vi "Spectrometer Control Panel (No Objects).vi"(8 "error in (no error)":errorcluster) -> (0 "error out":errorcluster)   [LabVIEW 2012]
uses:
  JY-SPEX-TRIAX/controls.llb/Turret Position (TRIAX).ctl
  JY-SPEX-TRIAX/controls.llb/Monochromator System Number.ctl
  JY-SPEX-TRIAX/controls.llb/Mirror Position.ctl
  Global/GPIB Type Def.ctl
  <vilib>/Utility/error.llb/DialogType.ctl
  JY-SPEX-TRIAX/controls.llb/Slits.ctl
  JY-SPEX-TRIAX/JY-SPEX-TRIAX.lvlib
panel:
  out "Shutter\nFunctional?":bool
  in  "JY Spectrometer":T1={"Name"="JY Spectrometer", "bus"=0.0, "GPIB"=1.0, "GPIB as string"="1", "byte"=1024, "VISA Resource Name"="GPIB0::1::INSTR"}
  out "Cluster Out":T5
  in  "Cluster In":T5
  out "?":bool
  out "Title 2":string="Spectrometer Control Program"
  in  "Select Grating":T4
  out "Construct":bool
  out "Init":T6
  out "Status":string
  in  "Shutter":bool
  in  "Set Mirror":bool
  in  "Exit Mirror Pos":bool=TRUE
  in  "Exit":bool
  out "Ready (when flashing)":bool
  out "Slits Open?":bool
  in  "Close Slits":bool
  in  "stepsize":dbl[unit]
  in  "Optimize":bool
  out "groovedensity":dbl[unit] caption="Groove Density"
  out "blazewave":dbl[unit] caption="Blaze Wavelength"
  in  "Set Turret":bool
  out "Title":string="Spectrometer Control Program"
  in  "Reset":bool
  out "Current Wavelength":dbl[unit]
  in  "Target Wavelength":dbl[unit]=4.0000000000000003e-07 min=0.0 max=1.4000000000000001e-06 step=1.0000000000000002e-10
  in  "Jump To Wavelength":bool
  in  "Set Slits":bool
  out "currentlat":dbl[unit] format="%#_6f"
  out "currentaxial":dbl[unit] format="%#_6f"
  in  "gotolat":dbl[unit] min=0.0 max=0.0022 step=1e-05
  in  "gotoaxial":dbl[unit] min=0.0 max=0.0022 step=1e-05 format="%#_6f"
  # "Initialization"
  # "Wavelength Control"
  # "Slit Widths"
  # "Turret and Other Specs"
  # "Target"
  # "Current"
  # "AXIAL/CCD"
  # "LATERAL/PMT"
  # "Axial Entrance"
  # "Lateral Exit"
  # "(will round to nearest step size - 2 µm)"
  # "Grooves/mm       Blaze           Cal Offset\nGrating A           1200           500 nm            -35571\nGrating B           1200           750 nm            -38317\nGrating C           Blank             N/A               -40000"
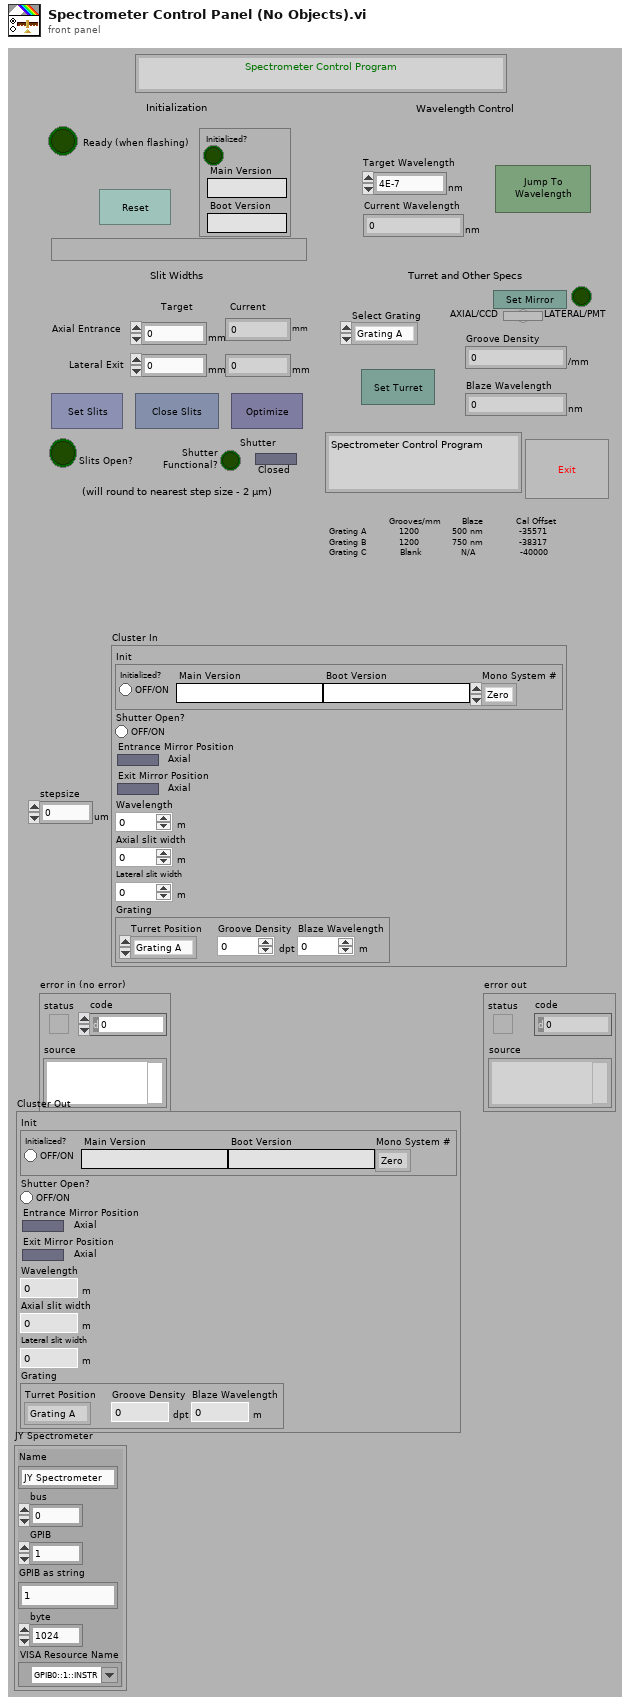
[diagram p1: front panel]
types:
  T1 = typedef "GPIB Type Def.ctl" = cluster{"Name":string, "bus":dbl, "GPIB":dbl, "GPIB as string":string, "byte":i32, "VISA Resource Name":refnum<visa-resource-name>}
  T2 = typedef "JY-SPEX-TRIAX.lvlib/Monochromator System Number.ctl" = enum16{"Zero", "One"}
  T3 = typedef "JY-SPEX-TRIAX.lvlib/Mirror Position.ctl" = bool
  T4 = typedef "JY-SPEX-TRIAX.lvlib/Turret Position (TRIAX).ctl" = enum16{"Grating A", "Grating B", "Grating C"}
  T5 = cluster{"Init":cluster{"Initialized?":bool, "Main Version":string, "Boot Version":string, "Mono System #":T2}, "Shutter Open?":bool, "Entrance Mirror Position":T3, "Exit Mirror Position":T3, "Wavelength":dbl[unit], "Axial slit width":dbl[unit], "Lateral slit width":dbl[unit], "Grating":cluster{"Turret Position":T4, "Groove Density":dbl[unit], "Blaze Wavelength":dbl[unit]}}
  T6 = cluster{"Initialized?":bool, "Main Version":string, "Boot Version":string, "Spectrometer Number":enum16{"Zero", "One"}}
  T7 = typedef "JY-SPEX-TRIAX.lvlib/Slits.ctl" = enum16{"0 (Front/Axial Entrance)", "1 (Side/Lateral Entrance)", "2 (Front/Axial Exit)", "3 (Side/Lateral Exit)"}
  T8 = typedef "DialogType.ctl" = u16
  T9 = cluster{"Initialized?":bool, "Main Version":string, "Boot Version":string, "Mono System #":T2}
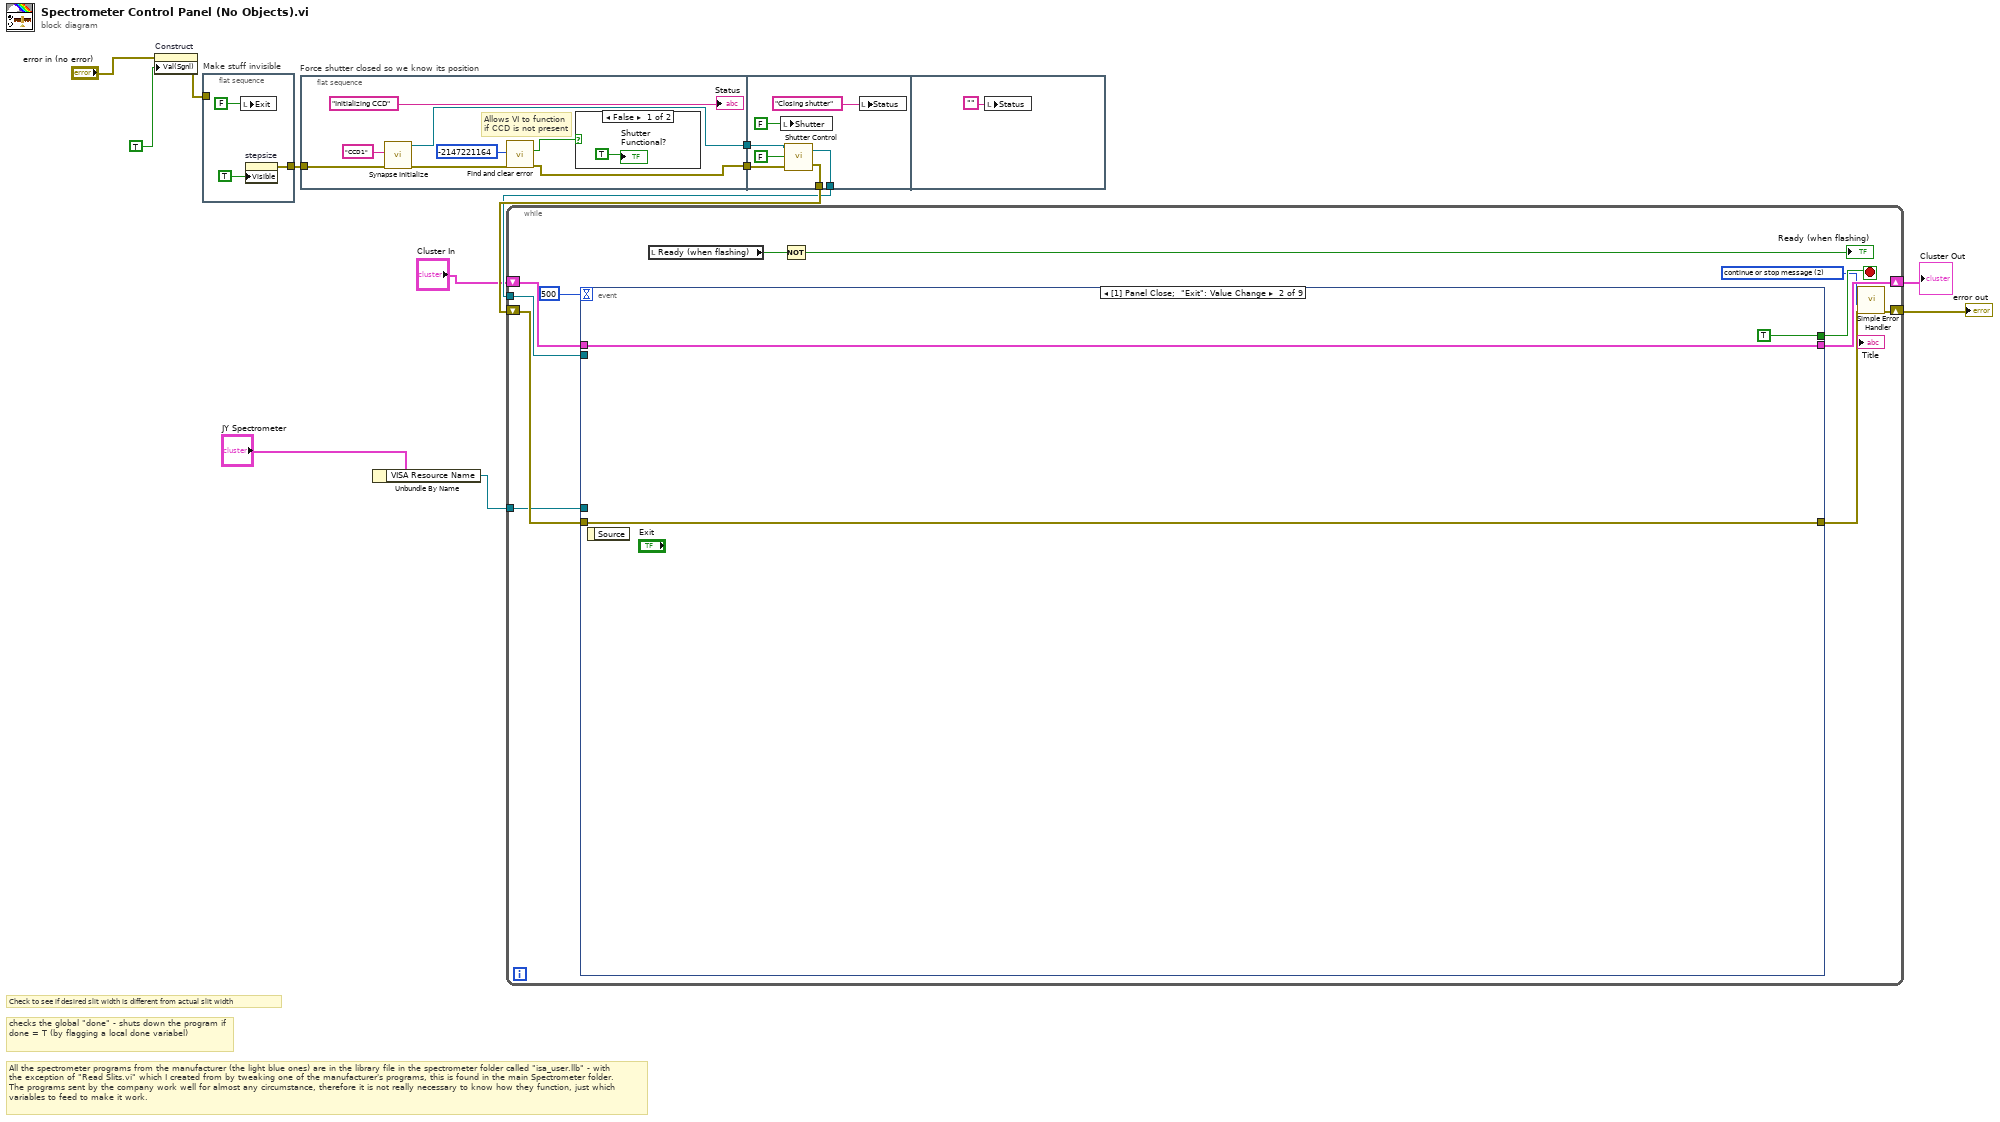
[diagram p0: block diagram]
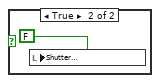
[diagram p2: hidden frame]
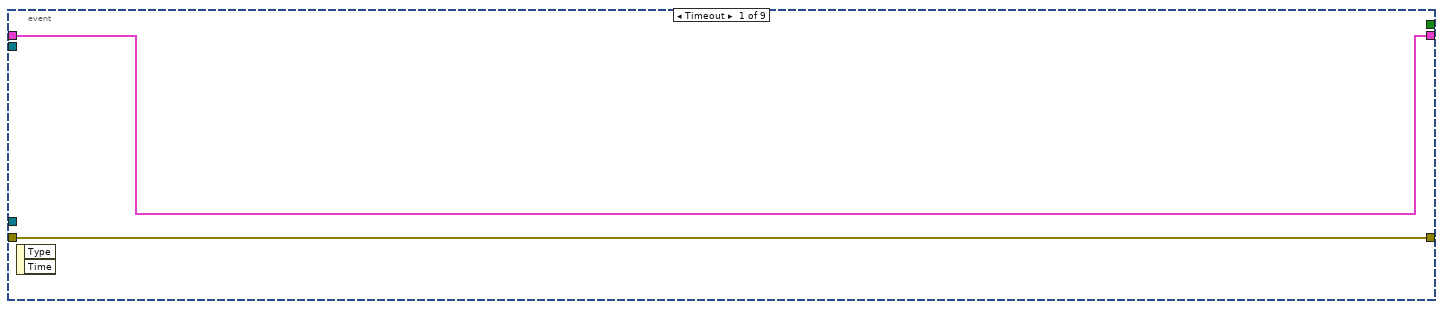
[diagram p3: hidden frame]
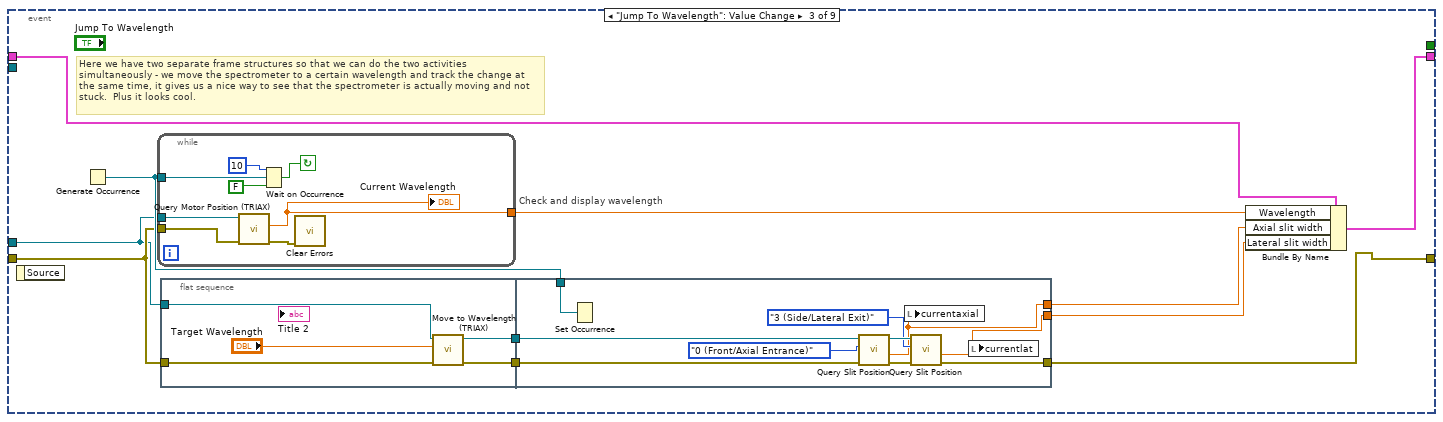
[diagram p4: hidden frame]
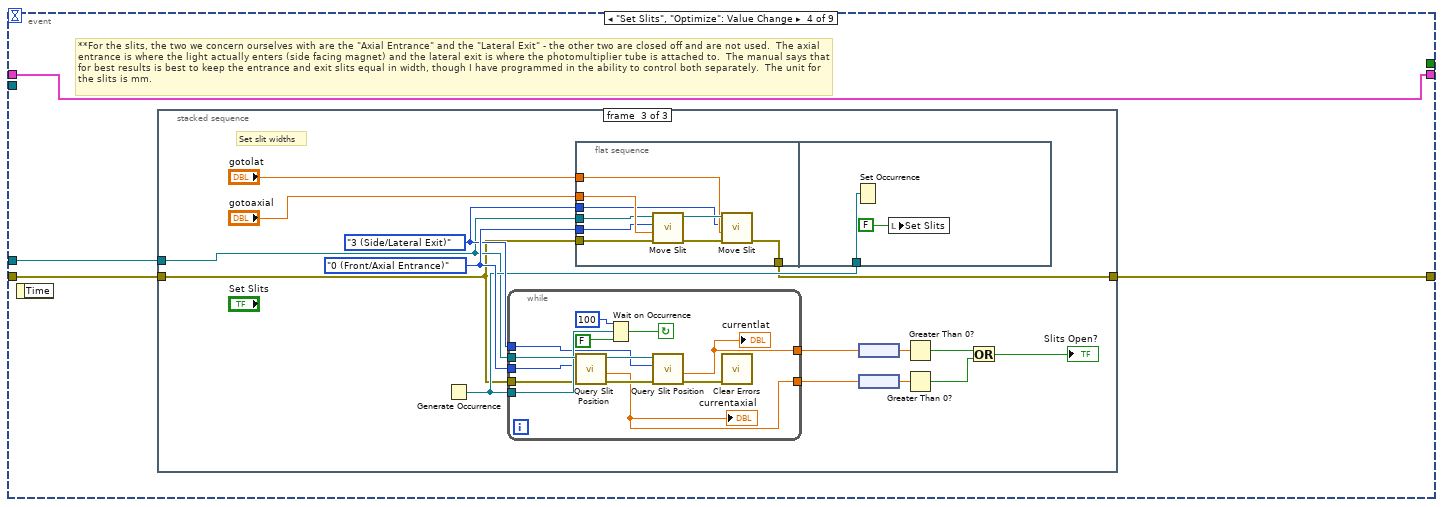
[diagram p5: hidden frame]
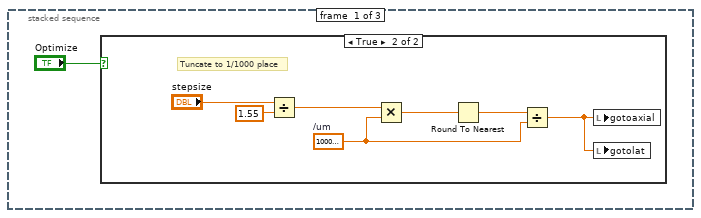
[diagram p6: hidden frame]
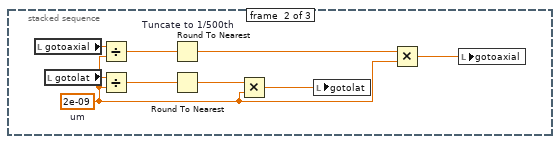
[diagram p8: hidden frame]
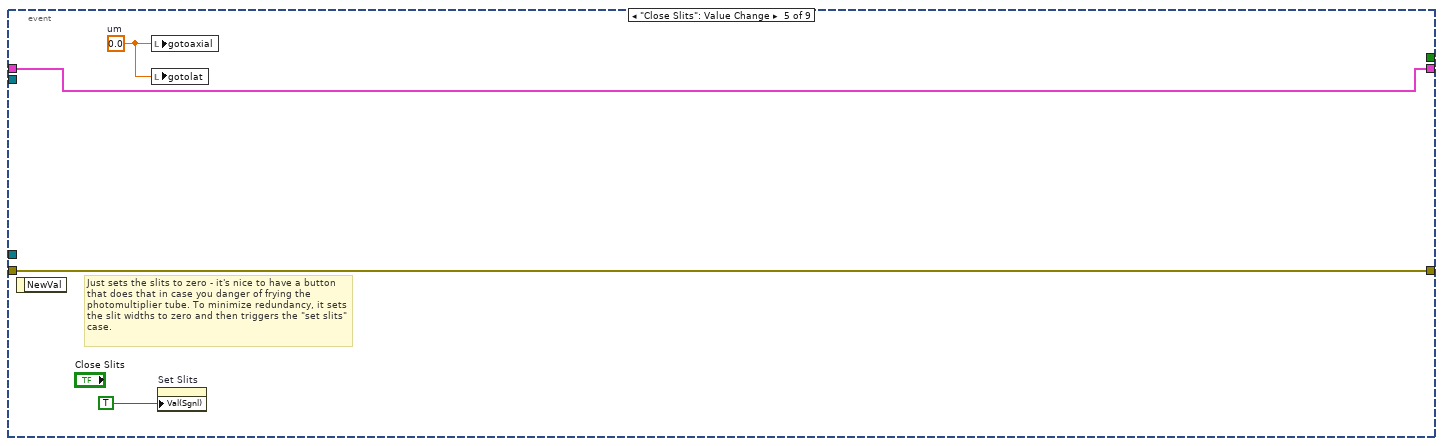
[diagram p9: hidden frame]
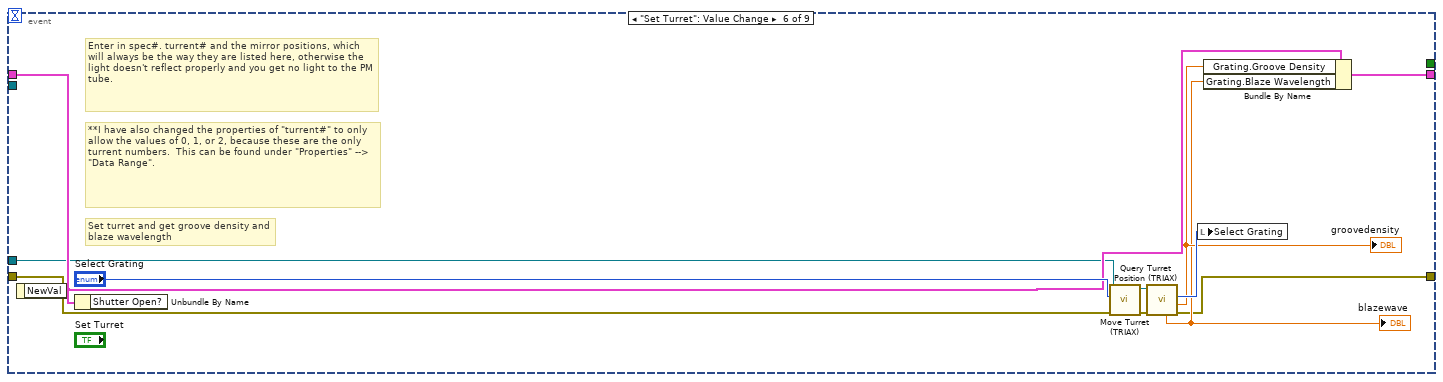
[diagram p10: hidden frame]
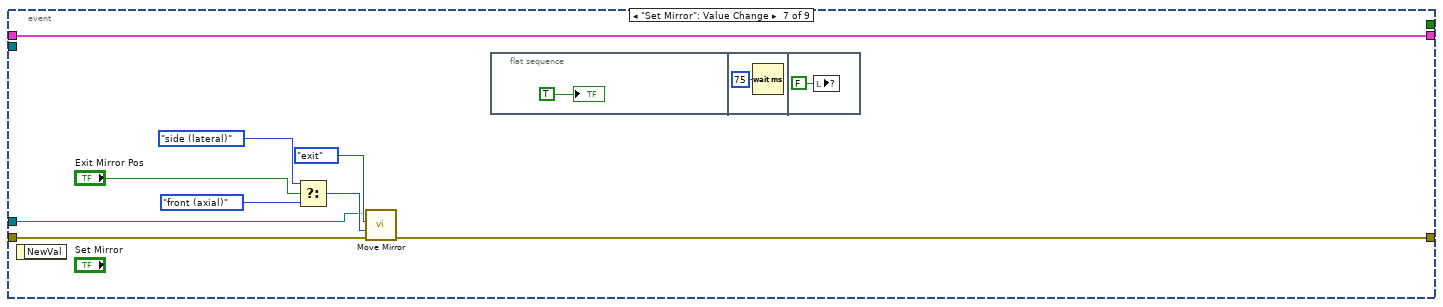
[diagram p11: hidden frame]
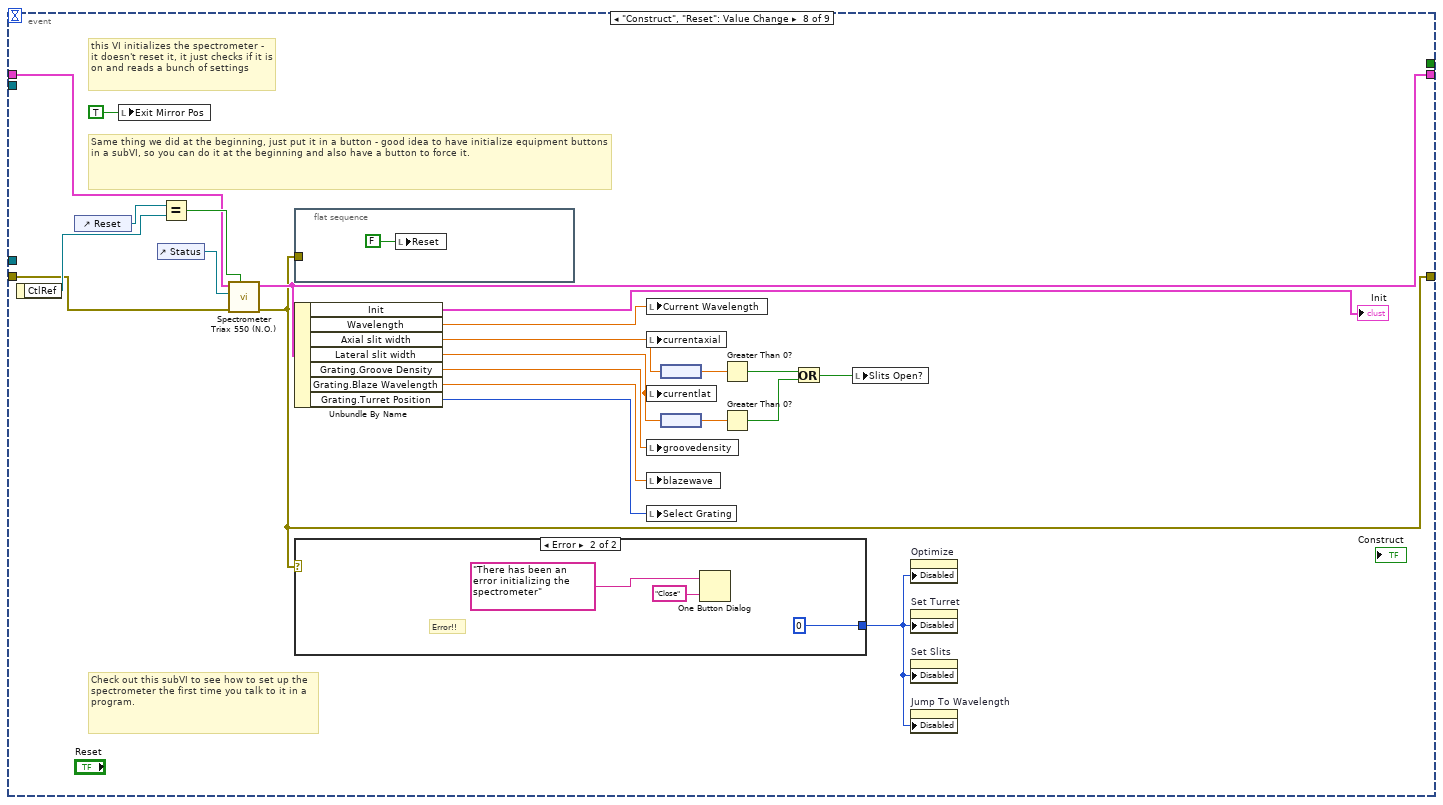
[diagram p12: hidden frame]
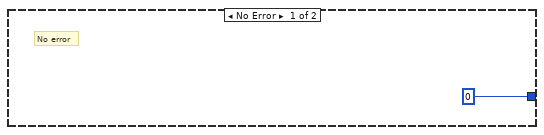
[diagram p13: hidden frame]
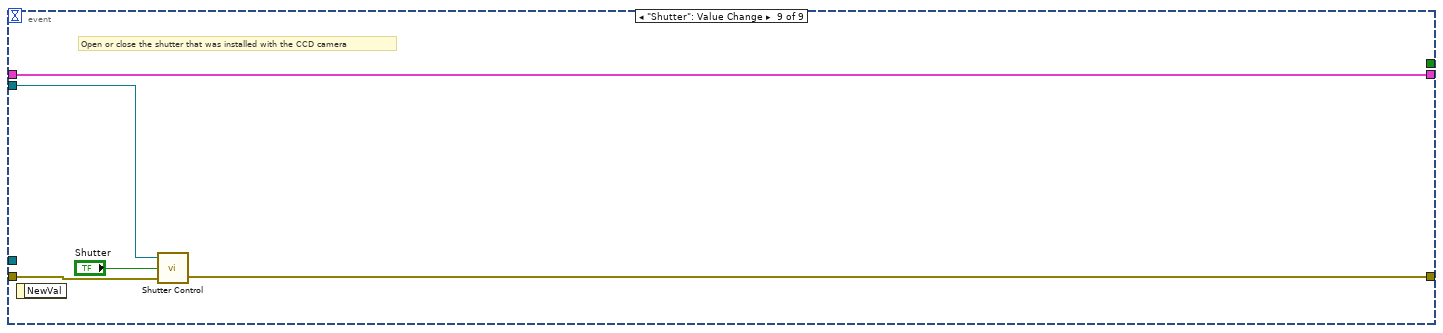
[diagram p14: hidden frame]
diagram:
  # "Check to see if desired slit width is different from actual slit width"
  # "checks the global \"done\" - shuts down the program if done = T (by flagging a local done variabel)"
  # "All the spectrometer programs from the manufacturer (the light blue ones) are in the library file in the spectrometer folder called \"isa_user.llb\" - with the exception of \"Read Slits.vi\" which I created from by tweaking one of the manufacturer's programs, this is found in the main Spectrometer folder.  The programs sent by the company work well for almost any circumstance, therefore it is not really necessary to know how they function, just which variables to feed to make it work."
  n1 = property on="Construct" class="Bool (strict)"(error in="error in (no error)", "Val(Sgnl)"=TRUE ("Value (Signaling)")) -> (error out=w12:errorcluster)  [unwired: 1 in, 1 out]
  n2 = flat-sequence "Make stuff invisible" {
    tunnel: w12 -> [_]
    tunnel: [w15] -> w9
    frame #0 {
      n3 = local write "Exit"(FALSE ("exit")) -> ()
      n4 = property on="stepsize" class="DigNum (strict)"("Visible"=TRUE) -> (error out=w15:errorcluster)  [unwired: 2 in, 1 out]
    }
  }
  n5 = flat-sequence "Force shutter closed so we know its position" {
    tunnel: w9 -> [w23]
    tunnel: [w18] -> w8
    tunnel: [w17] -> w1
    tunnel: [w31] -> w11
    tunnel: [w30] -> w10
    tunnel: w8 -> [w29]
    tunnel: w1 -> [w28]
    frame #0 {
      # "Allows VI to function\nif CCD is not present"
      n6 = call "Synapse Initialize.vi"("error in (no error)"=w23, "Unique id"="CCD1") -> ("error out"=w19:errorcluster, "JYCCDLib.IJYCCDReqd"=w17:refnum<k7>)  [unwired: 1 in, 7 out]
      n7 = call "Find and clear error.vi"("error in (no error)"=w19, "error code"=-2147221164) -> ("error out"=w18:errorcluster, "error found?"=w20:bool)  [unwired: 8 in]
      n8 = case shown="False" w20 {
        frame False {
          "Shutter\nFunctional?" <- TRUE
        }
        frame True {
          n9 = local write "Shutter\nFunctional?"(FALSE) -> ()
        }
      }
      "Status" <- "Initializing CCD" ("initialization progress")
    }
    frame #1 {
      n10 = local write "Shutter"(FALSE ("shutter")) -> ()
      n11 = call "Shutter Control.vi"("input error"=w29, "Shutter"=FALSE, "JYCCDLib.IJYCCDReqd"=w28) -> ("error out"=w31:errorcluster, "JYCCDLib.IJYCCDReqd 2"=w30:refnum<k7>)
      n12 = local write "Status"("Closing shutter" ("initialization progress")) -> ()
    }
    frame #2 {
      n13 = local write "Status"("") -> ()
    }
  }
  n14 = Unbundle By Name("JY Spectrometer") -> ("VISA Resource Name"=w5:refnum<visa-resource-name>)
  n15 = while {
    tunnel: w10 -> [w38]
    shift-right: [w40] -> w3
    shift-left: "Cluster In" -> [w42]
    shift-right: [w37] -> w4
    shift-left: w11 -> [w41]
    tunnel: w5 -> [w35]
    stop <- w46 stop-if-true
    w36 = T8 2 items=["no dialog", "OK message", "continue or stop message", "OK message + warnings", "continue/stop + warnings"] ("type of dialog (OK msg:1)")
    n16 = event shown="[1] Panel Close;  \"Exit\": Value Change" {
      selector: _ -> [_ _ _ _ _ _ _ _ _]
      dyn-events: _ -> [_ _ _ _ _ _ _ _ _]
      timeout: 500 -> [_ _ _ _ _ _ _ _ _]
      tunnel: [_ TRUE _ _ _ _ _ _ _] -> w46
      tunnel: w38 -> [_ _ _ _ _ _ _ _ w204]
      tunnel: [w47 w50 w52 w87 w148 w160 w161 w182 w202] -> w40
      tunnel: w42 -> [w47 w50 w56 w87 w148 w153 w161 w173 w202]
      tunnel: [w48 w49 w53 w86 w146 w152 w164 w180 w200] -> w39
      tunnel: w41 -> [w48 w49 w55 w88 w146 w151 w163 w174 w201]
      tunnel: w35 -> [_ _ w54 w89 _ w150 w162 _ _]
      event Timeout {
        n17 = event-data() -> ()  [unwired: 3 out]
      }
      event Panel Close; "Exit": Value Change {
        n18 = event-data() -> ()  [unwired: 2 out]
      }
      event "Jump To Wavelength": Value Change {
        # "Here we have two separate frame structures so that we can do the two activities simultaneously - we move the spectrometer to a certain wavelength and track the change at the same time, it gives us a nice way to see that the spectrometer is actually moving and not stuck.  Plus it looks cool."
        n19 = event-data() -> ()  [unwired: 2 out]
        n20 = Generate Occurrence() -> (w59:refnum<k4>)
        n21 = while "Check and display wavelength" {
          tunnel: [w78] -> w62
          tunnel: w59 -> [w83]
          tunnel: w54 -> [w81]
          tunnel: w55 -> [w79]
          stop <- w85 continue-if-true
          n22 = call "Query Motor Position (TRIAX).vi"("error in (no error)"=w79, "VISA resource name"=w81) -> ("error out"=w80:errorcluster, "wavelength"=w78:dbl[unit])  [unwired: 1 in, 7 out]
          "Current Wavelength" <- w78
          n23 = Wait on Occurrence(1:FALSE ("ignore previous (T)"), 2:w83, 3:10 ("ms timeout (-1)")) -> (0:w85:bool)
          n24 = call <vilib>:"Clear Errors.vi"("error in (no error)"=w80) -> ()  [unwired: 7 out]
        }
        n25 = flat-sequence {
          tunnel: w54 -> [w67]
          tunnel: [w66] -> w58
          tunnel: [w65] -> w57
          tunnel: w55 -> [w64]
          tunnel: [w68] -> w61
          tunnel: [w72] -> w60
          tunnel: w59 -> [w77]
          tunnel: w58 -> [w75]
          tunnel: w57 -> [w74]
          tunnel: [w70] -> w53
          frame #0 {
            n26 = call "Move to Wavelength (TRIAX).vi"("error in (no error)"=w64, "Target wavelength"="Target Wavelength", "VISA resource name"=w67) -> ("error out"=w65:errorcluster, "VISA resource name out"=w66:refnum<visa-resource-name>)  [unwired: 1 in, 6 out]
          }
          frame #1 {
            n27 = Set Occurrence(w77) -> ()
            n28 = call "Query Slit Position.vi"("error in (no error)"=w74, "Slit (Front/Axial Entrance)"=Slits."0 (Front/Axial Entrance)", "VISA resource name"=w75) -> ("error out"=w69:errorcluster, "Slit Position"=w68:dbl[unit], "VISA resource name out"=w76:refnum<visa-resource-name>)  [unwired: 1 in, 5 out]
            n29 = local write "currentaxial"(w68) -> ()
            n30 = call "Query Slit Position.vi"("error in (no error)"=w69, "Slit (Front/Axial Entrance)"=Slits."3 (Side/Lateral Exit)", "VISA resource name"=w76) -> ("error out"=w70:errorcluster, "Slit Position"=w72:dbl[unit])  [unwired: 1 in, 6 out]
            n31 = local write "currentlat"(w72) -> ()
          }
        }
        n32 = Bundle By Name(cluster=w56, "Wavelength"=w62, "Axial slit width"=w61, "Lateral slit width"=w60) -> (w52:T5)
      }
      event "Set Slits", "Optimize": Value Change {
        # "**For the slits, the two we concern ourselves with are the \"Axial Entrance\" and the \"Lateral Exit\" - the other two are closed off and are not used.  The axial entrance is where the light actually enters (side facing magnet) and the lateral exit is where the photomultiplier tube is attached to.  The manual says that for best results is best to keep the entrance and exit slits equal in width, though I have programmed in the ability to control both separately.  The unit for the slits is mm."
        n33 = event-data() -> ()  [unwired: 2 out]
        n34 = stacked-sequence {
          tunnel: [_ _ w109] -> w86
          tunnel: w88 -> [_ _ w107]
          tunnel: w89 -> [_ _ w108]
          frame #0 {
            n35 = case shown="True" "Optimize" {
              frame False {
              }
              frame True {
                w95 = dbl[unit] 1000000000.0  # /um
                # "Tuncate to 1/1000 place"
                n36 = Divide(x="stepsize", y=1.55) -> (x/y=w97:dbl[unit])
                n37 = Multiply(x=w97, y=w95) -> (x*y=w96:dbl)
                n38 = Round To Nearest(number=w96) -> (nearest integer value=w94:dbl)
                n39 = Divide(x=w94, y=w95) -> (x/y=w91:dbl[unit])
                n40 = local write "gotoaxial"(w91) -> ()
                n41 = local write "gotolat"(w91) -> ()
              }
            }
          }
          frame #1 {
            w102 = dbl[unit] 2e-09  # um
            n42 = local read "gotoaxial"() -> (w104:dbl[unit])
            n43 = local read "gotolat"() -> (w103:dbl[unit])
            n44 = Divide(x=w104, y=w102) -> (x/y=w101:dbl)
            n45 = Divide(x=w103, y=w102) -> (x/y=w99:dbl)
            n46 = Round To Nearest "Tuncate to 1/500th"(number=w101) -> (nearest integer value=w100:dbl)
            n47 = Round To Nearest(number=w99) -> (nearest integer value=w98:dbl)
            n48 = Multiply(x=w98, y=w102) -> (x*y=w105:dbl[unit])
            n49 = local write "gotolat"(w105) -> ()
            n50 = Multiply(x=w100, y=w102) -> (x*y=w106:dbl[unit])
            n51 = local write "gotoaxial"(w106) -> ()
          }
          frame #2 {
            w111 = Slits."3 (Side/Lateral Exit)" ("Slit (Front/Axial Entrance)")
            w112 = Slits."0 (Front/Axial Entrance)" ("Slit (Front/Axial Entrance)")
            # "Set slit widths"
            n52 = Generate Occurrence() -> (w110:refnum<k4>)
            n53 = while {
              tunnel: w108 -> [w144]
              tunnel: [w141] -> w114
              tunnel: [w140] -> w113
              tunnel: w110 -> [w139]
              tunnel: w107 -> [w136]
              tunnel: w112 -> [w135]
              tunnel: w111 -> [w134]
              stop <- w137 continue-if-true
              n54 = call "Query Slit Position.vi"("error in (no error)"=w136, "Slit (Front/Axial Entrance)"=w135, "VISA resource name"=w144) -> ("error out"=w143:errorcluster, "Slit Position"=w141:dbl[unit], "VISA resource name out"=w145:refnum<visa-resource-name>)  [unwired: 1 in, 5 out]
              "currentaxial" <- w141
              n55 = Wait on Occurrence(1:FALSE ("ignore previous (T)"), 2:w139, 3:100 ("ms timeout (-1)")) -> (0:w137:bool)
              n56 = call "Query Slit Position.vi"("error in (no error)"=w143, "Slit (Front/Axial Entrance)"=w134, "VISA resource name"=w145) -> ("error out"=w142:errorcluster, "Slit Position"=w140:dbl[unit])  [unwired: 1 in, 6 out]
              "currentlat" <- w140
              n57 = call <vilib>:"Clear Errors.vi"("error in (no error)"=w142) -> ()  [unwired: 7 out]
            }
            n58 = flat-sequence {
              tunnel: "gotoaxial" -> [w129]
              tunnel: "gotolat" -> [w128]
              tunnel: w108 -> [w126]
              tunnel: w107 -> [w125]
              tunnel: w112 -> [w124]
              tunnel: w111 -> [w123]
              tunnel: [w122] -> w109
              tunnel: w110 -> [w132]
              frame #0 {
                n59 = call "Move Slit.vi"("error in (no error)"=w125, "Desired Slit Position"=w129, "Slit (Front/Axial Entrance)"=w124, "VISA resource name"=w126) -> ("error out"=w127:errorcluster, "VISA resource name out"=w130:refnum<visa-resource-name>)  [unwired: 1 in, 5 out]
                n60 = call "Move Slit.vi"("error in (no error)"=w127, "Desired Slit Position"=w128, "Slit (Front/Axial Entrance)"=w123, "VISA resource name"=w130) -> ("error out"=w122:errorcluster)  [unwired: 1 in, 6 out]
              }
              frame #1 {
                n61 = Set Occurrence(w132) -> ()
                n62 = local write "Set Slits"(FALSE ("Move Slits")) -> ()
              }
            }
            n63 = node(w113) -> (w121:dbl)
            n64 = node(w114) -> (w120:dbl)
            n65 = Greater Than 0?(x=w121) -> (x > 0?=w117:bool)
            n66 = Greater Than 0?(x=w120) -> (x > 0?=w118:bool)
            n67 = Or(x=w117, y=w118) -> (x .or. y?=→"Slits Open?":bool)
          }
        }
      }
      event "Close Slits": Value Change {
        w149 = dbl[unit] 0.0  # um
        # "Just sets the slits to zero - it's nice to have a button that does that in case you danger of frying the photomultiplier tube. To minimize redundancy, it sets the slit widths to zero and then triggers the \"set slits\" case."
        n68 = event-data() -> ()  [unwired: 2 out]
        n69 = local write "gotoaxial"(w149) -> ()
        n70 = local write "gotolat"(w149) -> ()
        n71 = property on="Set Slits" class="Bool (strict)"("Val(Sgnl)"=TRUE ("Value (Signaling)")) -> ()  [unwired: 2 in, 2 out]
      }
      event "Set Turret": Value Change {
        # "**I have also changed the properties of \"turrent#\" to only allow the values of 0, 1, or 2, because these are the only turrent numbers.  This can be found under \"Properties\" --> \"Data Range\"."
        # "Enter in spec#. turrent# and the mirror positions, which will always be the way they are listed here, otherwise the light doesn't reflect properly and you get no light to the PM tube."
        # "Set turret and get groove density and \nblaze wavelength"
        n72 = event-data() -> ()  [unwired: 2 out]
        n73 = Unbundle By Name(w153) -> ()  [unwired: 1 out]
        n74 = call "Move Turret (TRIAX).vi"("error in (no error)"=w151, "turret position (0)"="Select Grating", "VISA resource name"=w150) -> ("error out"=w157:errorcluster, "VISA resource name out"=w158:refnum<visa-resource-name>)  [unwired: 1 in, 6 out]
        n75 = call "Query Turret Position (TRIAX).vi"("error in (no error)"=w157, "VISA resource name"=w158) -> ("error out"=w152:errorcluster, "Groove Density"=w155:dbl[unit], "Turret Position"=w156:T4, "Blaze Wavelength"=w154:dbl[unit])  [unwired: 1 in, 5 out]
        "blazewave" <- w154
        "groovedensity" <- w155
        n76 = local write "Select Grating"(w156) -> ()
        n77 = Bundle By Name(cluster=w153, "Grating.Groove Density"=w155, "Grating.Blaze Wavelength"=w154) -> (w160:T5)
      }
      event "Set Mirror": Value Change {
        n78 = event-data() -> ()  [unwired: 2 out]
        n79 = Select(t=enum16{"side (lateral)", "front (axial)"}."side (lateral)" ("position (side/lateral)"), s="Exit Mirror Pos", f=enum16{"side (lateral)", "front (axial)"}."front (axial)" ("position (side/lateral)")) -> (s? t:f=w165:enum16{"side (lateral)", "front (axial)"})
        n80 = call "Move Mirror.vi"("error in (no error)"=w163, "position (side/lateral)"=w165, "mirror (exit)"=enum16{"entrance", "exit"}."exit", "VISA resource name"=w162) -> ("error out"=w164:errorcluster)  [unwired: 1 in, 6 out]
        n81 = flat-sequence {
          frame #0 {
            "?" <- TRUE ("Mirror set")
          }
          frame #1 {
            n82 = Wait (ms)(milliseconds to wait=u32 75) -> ()  [unwired: 1 out]
          }
          frame #2 {
            n83 = local write item#29(FALSE ("Mirror set")) -> ()
          }
        }
      }
      event "Construct", "Reset": Value Change {
        # "Check out this subVI to see how to set up the spectrometer the first time you talk to it in a program."
        # "this VI initializes the spectrometer - it doesn't reset it, it just checks if it is on and reads a bunch of settings"
        # "Same thing we did at the beginning, just put it in a button - good idea to have initialize equipment buttons in a subVI, so you can do it at the beginning and also have a button to force it."
        n84 = event-data() -> ("CtlRef"=w177:refnum<vi>)  [unwired: 1 out]
        n85 = control-ref of="Reset"() -> (w176:refnum<vi>)
        n86 = local write "Exit Mirror Pos"(TRUE ("Exit Mirror Pos")) -> ()
        n87 = control-ref of="Status"() -> (w179:refnum<vi>)
        n88 = Equal?(x=w176, y=w177) -> (x = y?=w175:bool)
        n89 = call "Spectrometer Triax 550 (N.O.).vi"("Force Reset? (F)"=w175, "error in (no error)"=w174, "Ref to a Status Box"=w179, "Cluster In"=w173) -> ("error out"=w180:errorcluster, "Cluster Out"=w182:T5)  [unwired: 6 in]
        n90 = flat-sequence {
          tunnel: w180 -> [_]
          frame #0 {
            n91 = local write "Reset"(FALSE ("initialize")) -> ()
          }
        }
        n92 = Unbundle By Name(w182) -> ("Init"=→"Init":T9, "Wavelength"=w190:dbl[unit], "Axial slit width"=w183:dbl[unit], "Lateral slit width"=w187:dbl[unit], "Grating.Groove Density"=w189:dbl[unit], "Grating.Blaze Wavelength"=w188:dbl[unit], "Grating.Turret Position"=w181:T4)
        n93 = case shown="Error" w180 {
          tunnel: [0 0] -> w194
          frame No Error {
            # "No error"
          }
          frame Error {
            # "Error!!"
            n94 = One Button Dialog(message="There has been an error initializing the spectrometer", button name ("OK")="Close") -> ()  [unwired: 1 out]
          }
        }
        n95 = local write "Current Wavelength"(w190) -> ()
        n96 = local write "currentaxial"(w183) -> ()
        n97 = local write "currentlat"(w187) -> ()
        n98 = local write "groovedensity"(w189) -> ()
        n99 = local write "blazewave"(w188) -> ()
        n100 = local write "Select Grating"(w181) -> ()
        n101 = node(w183) -> (w185:dbl)
        n102 = node(w187) -> (w184:dbl)
        n103 = Greater Than 0?(x=w185) -> (x > 0?=w193:bool)
        n104 = Greater Than 0?(x=w184) -> (x > 0?=w192:bool)
        n105 = Or(x=w193, y=w192) -> (x .or. y?=w191:bool)
        n106 = local write "Slits Open?"(w191) -> ()
        n107 = property on="Optimize" class="Bool"("Disabled"=w194) -> ()  [unwired: 2 in, 2 out]
        n108 = property on="Set Turret" class="Bool"("Disabled"=w194) -> ()  [unwired: 2 in, 2 out]
        n109 = property on="Set Slits" class="Bool (strict)"("Disabled"=w194) -> ()  [unwired: 2 in, 2 out]
        n110 = property on="Jump To Wavelength" class="Bool"("Disabled"=w194) -> ()  [unwired: 2 in, 2 out]
      }
      event "Shutter": Value Change {
        # "Open or close the shutter that was installed with the CCD camera"
        n111 = event-data() -> ()  [unwired: 2 out]
        n112 = call "Shutter Control.vi"("input error"=w201, "Shutter"="Shutter", "JYCCDLib.IJYCCDReqd"=w204) -> ("error out"=w200:errorcluster)  [unwired: 1 out]
      }
    }
    n113 = local read "Ready (when flashing)"() -> (w44:bool)
    n114 = Not(x=w44) -> (.not. x?=→"Ready (when flashing)":bool)
    n115 = call <vilib>:"Simple Error Handler.vi"("type of dialog (OK msg:1)"=w36, "error in (no error)"=w39) -> ("error out"=w37:errorcluster)  [unwired: 7 out]
  }
  "error out" <- w4
  "Cluster Out" <- w3
